vi "Set-control-variant.vi"(8 "error in (no error)":errorcluster, 9 "Value":variant, 10 "Control name":T1, 11 "Panes in":T2) -> (0 "error out":errorcluster, 3 "Panes out":T2)   [LabVIEW 2013, in "MaterialCharacterization.lvlib" / "MC-UI.lvclass"]
uses:
  MC-UI.lvclass
  Panes-reference.ctl
  Control-names.ctl
  MC-UI.lvclass/MC-UI.ctl
  Read Controls lib.vi
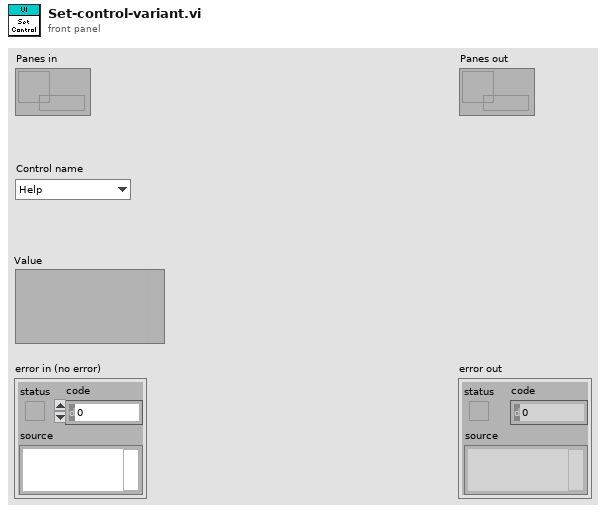
[diagram p1: front panel]
types:
  T1 = typedef "MaterialCharacterization.lvlib/MC-UI.lvclass/Control-names.ctl" = enum16{"Help", "Status", "Load configuration", "Save configuration", "Activate", "Start", "Stop", "Options"}
  T2 = typedef "MaterialCharacterization.lvlib/MC-UI.lvclass/Panes-reference.ctl" = refnum<data-value>
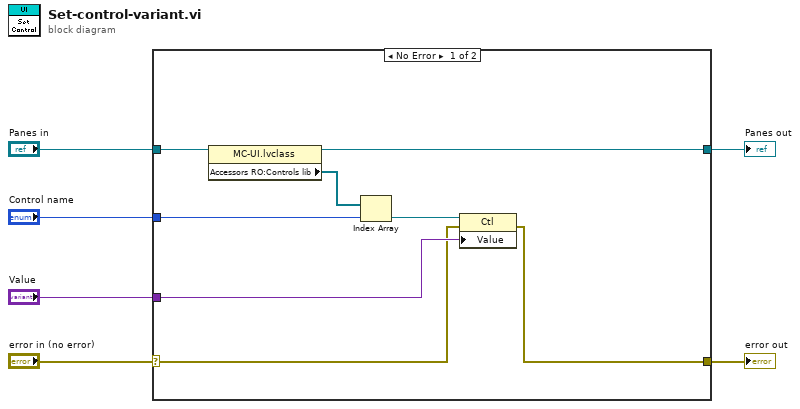
[diagram p0: block diagram]
diagram:
  n1 = case shown="No Error" "error in (no error)" {
    selector: "error in (no error)" -> [w9 w15]
    tunnel: [w8 w15] -> w5
    tunnel: [w7 w16] -> w3
    tunnel: "Panes in" -> [w14 w16]
    tunnel: "Control name" -> [w12 _]
    tunnel: "Value" -> [w10 _]
    frame No Error {
      n2 = property class="MC-UI.lvclass"(reference=w14) -> (reference out=w7:T2, "Accessors RO:Controls lib"=w13:refnum<vi>[])  [unwired: 1 in, 1 out]
      n3 = Index Array(array=w13, index=w12) -> (element=w11:refnum<vi>)
      n4 = property class="Ctl"(reference=w11, error in=w9, "Value"=w10) -> (error out=w8:errorcluster)  [unwired: 1 out]
    }
    frame Error {
    }
  }
  "error out" <- w5
  "Panes out" <- w3
